vi "Create Delete Symbol Overlays_Cluster.vi"(11 "Tree Ref":refnum<vi>) -> ()   [LabVIEW 2023]
panel:
  in  "Tree":string[](tree)
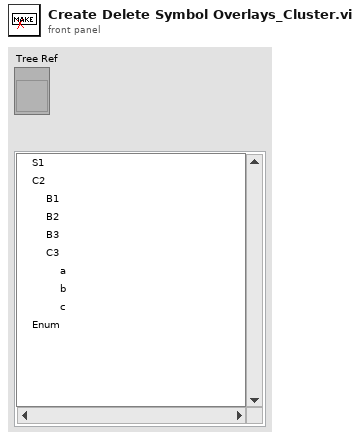
[diagram p1: front panel]
types:
  T1 = cluster{"left":i16, "top":i16, "right":i16, "bottom":i16}
  T2 = cluster{"image type":i32, "image depth":i32, "image":u8[], "mask":u8[], "colors":u32[], "Rectangle":cluster{"left":i16, "top":i16, "right":i16, "bottom":i16}}[]
  T3 = cluster{"image type":i32, "image depth":i32, "image":u8[], "mask":u8[], "colors":u32[], "Rectangle":cluster{"left":i16, "top":i16, "right":i16, "bottom":i16}}
  T4 = typedef "imagedata.ctl" = cluster{"image type":i32, "image depth":i32, "image":u8[], "mask":u8[], "colors":u32[], "Rectangle":cluster{"left":i16, "top":i16, "right":i16, "bottom":i16}}
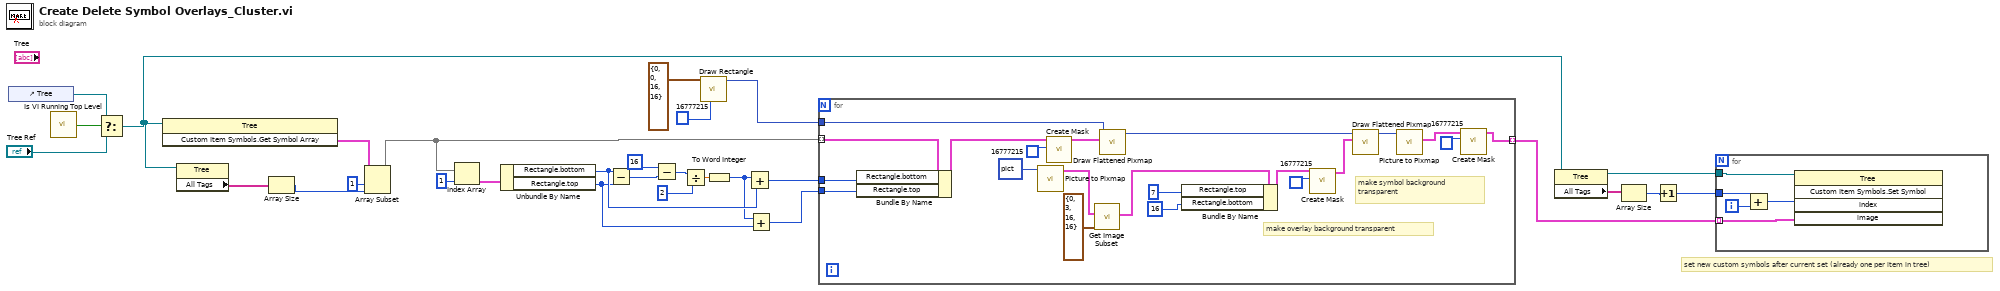
[diagram p0: block diagram]
diagram:
  # "set new custom symbols after current set (already one per item in tree)"
  n1 = control-ref of="Tree"() -> (w20:refnum<vi>)
  n2 = call "Is VI Running Top Level.vi"() -> ("Top Level?"=w21:bool)  [unwired: 5 in]
  n3 = Select(t=w20, s=w21, f="Tree Ref") -> (s? t:f=w6:refnum<vi>)
  n4 = invoke class="Tree" method="Custom Item Symbols.Get Symbol Array"(reference=w6) -> ("Custom Glyphs:Get Glyph Array"=w2:T2)  [unwired: 2 in, 2 out]
  n5 = property class="Tree"(reference=w6) -> ("All Tags"=w5:string[])  [unwired: 1 in, 2 out]
  n6 = Array Size(array=w5) -> (size(s)=w4:i32)
  n7 = Array Subset(array=w2, index=1, length=w4) -> (w1:T2)
  n8 = Index Array(array=w1, index=1) -> (element=w14:T3)
  n9 = Unbundle By Name(w14) -> ("Rectangle.bottom"=w13:i16, "Rectangle.top"=w12:i16)
  n10 = Subtract(x=w13, y=w12) -> (x-y=w15:i16)
  n11 = Subtract(x=i16 16 ("bottom"), y=w15) -> (x-y=w17:i16)
  n12 = Divide(x=w17, y=i16 2 ("bottom")) -> (x/y=w11:dbl)
  n13 = call <vilib>:"Draw Rectangle.vi"("rect"=T1 {"left"=0, "top"=0, "right"=16, "bottom"=16}, "color(black)"=u32 16777215) -> ("new picture"=w22:picture)  [unwired: 7 in]
  n14 = To Word Integer(number=w11) -> (16bit integer=w8:i16)
  n15 = Add(x=w8, y=w13) -> (x+y=w7:i16)
  n16 = Add(x=w8, y=w12) -> (x+y=w10:i16)
  n17 = for {
    tunnel: [w30] -> w28 mode=indexing
    tunnel: w1 -> [w43] mode=indexing
    tunnel: w22 -> [w46]
    tunnel: w7 -> [w45]
    tunnel: w10 -> [w44]
    # "make symbol background transparent"
    # "make overlay background transparent"
    n18 = Bundle By Name(cluster=w43, "Rectangle.bottom"=w45, "Rectangle.top"=w44) -> (w35:T3)
    n19 = call <vilib>:"Picture to Pixmap.vi"("picture"=picture bytes[830] ("new picture")) -> ("image data"=w41:T4)  [unwired: 9 in, 1 out]
    n20 = call <vilib>:"Create Mask.vi"("Mask Color (Black)"=u32 16777215, "image data"=w35) -> ("image data"=w34:T4)  [unwired: 9 in]
    n21 = call <vilib>:"Get Image Subset.vi"("subset rect"=T1 {"left"=0, "top"=3, "right"=16, "bottom"=16}, "image data"=w41) -> ("image subset"=w40:T4)  [unwired: 4 in, 1 out]
    n22 = call <vilib>:"Draw Flattened Pixmap.vi"("image data"=w34, "picture"=w46) -> ("new picture"=w49:picture)  [unwired: 7 in]
    n23 = Bundle By Name(cluster=w40, "Rectangle.top"=i16 7 ("left"), "Rectangle.bottom"=i16 16 ("left")) -> (w39:T4)
    n24 = call <vilib>:"Create Mask.vi"("Mask Color (Black)"=u32 16777215, "image data"=w39) -> ("image data"=w48:T4)  [unwired: 9 in]
    n25 = call <vilib>:"Draw Flattened Pixmap.vi"("image data"=w48, "picture"=w49) -> ("new picture"=w33:picture)  [unwired: 7 in]
    n26 = call <vilib>:"Picture to Pixmap.vi"("picture"=w33) -> ("image data"=w32:T4)  [unwired: 9 in, 1 out]
    n27 = call <vilib>:"Create Mask.vi"("Mask Color (Black)"=u32 16777215, "image data"=w32) -> ("image data"=w30:T4)  [unwired: 9 in]
  }
  n28 = property class="Tree"(reference=w6) -> (reference out=w27:refnum<vi>, "All Tags"=w25:string[])  [unwired: 1 in, 1 out]
  n29 = Array Size(array=w25) -> (size(s)=w26:i32)
  n30 = Increment(x=w26) -> (x+1=w29:i32)
  n31 = for {
    tunnel: w27 -> [w55]
    tunnel: w28 -> [w54] mode=indexing
    tunnel: w29 -> [w53]
    i -> [w52]
    n32 = Add(x=w53, y=w52) -> (x+y=w51:i32)
    n33 = invoke class="Tree" method="Custom Item Symbols.Set Symbol"(reference=w55, "index"=w51, "image"=w54) -> ()  [unwired: 2 in, 5 out]
  }
